vi "ElevatorSim_WouldHitUpperLimit.vi"(10 "Height_Meters":dbl=1.0, 11 "ElevatorSim":T1 {"GearBox"."Kt_NMPerAmp" format="%13.5p"; "GearBox"."Kv_RadPerSecPerVolt" format="%13.5p"; "GearBox"."R_Ohms" format="%13.5p"; "GearBox"."FreeSpeed_RadPerSec" format="%13.5p"; "GearBox"."FreeCurrent_Amps" format="%13.5p"; "GearBox"."StallCurrent_Amps" format="%13.5p"; "GearBox"."StallTorque_NM" format="%13.5p"; "GearBox"."nominalVoltage_Volts" format="%13.5p"}) -> (3 "At HIgh LImit":bool)   [LabVIEW 2019, in "Trajectory_Library.lvlib"]
doc: "Creates a new LINEAR SYSTEM data cluster with the specified values. \n\n\nInputs: \n - XXX -- XXX.\n\nOutputs:\n - XXX -- XXX."
uses:
  LinearSystem_New.vi
  MatBuilder_Create.vi
  MatBuilder_Fill.vi
  MatrixHelper_Zero.vi
  MatrixHelper_CoerceSize.vi
  Trajectory_Library.lvlib
  LINEAR_SYSTEM.ctl
  <vilib>/Analysis/Matrix/Datatypes/RealMatrix.ctl
  <vilib>/Analysis/Matrix/NI_Matrix.lvlib
  DCMOTOR.CTL
  LINEAR_SYSTEM_SIM.ctl
  ELEVATOR_SIM.ctl
panel:
  # "<States, 1>"
  # "<Outputs, 1>"
  # "<Inputs, 1>"
  # "<Outputs, 1>"
  # "<States,States>"
  # "<States,Inputs>"
  # "<Outputs,States>"
  # "<Outputs,Inputs>"
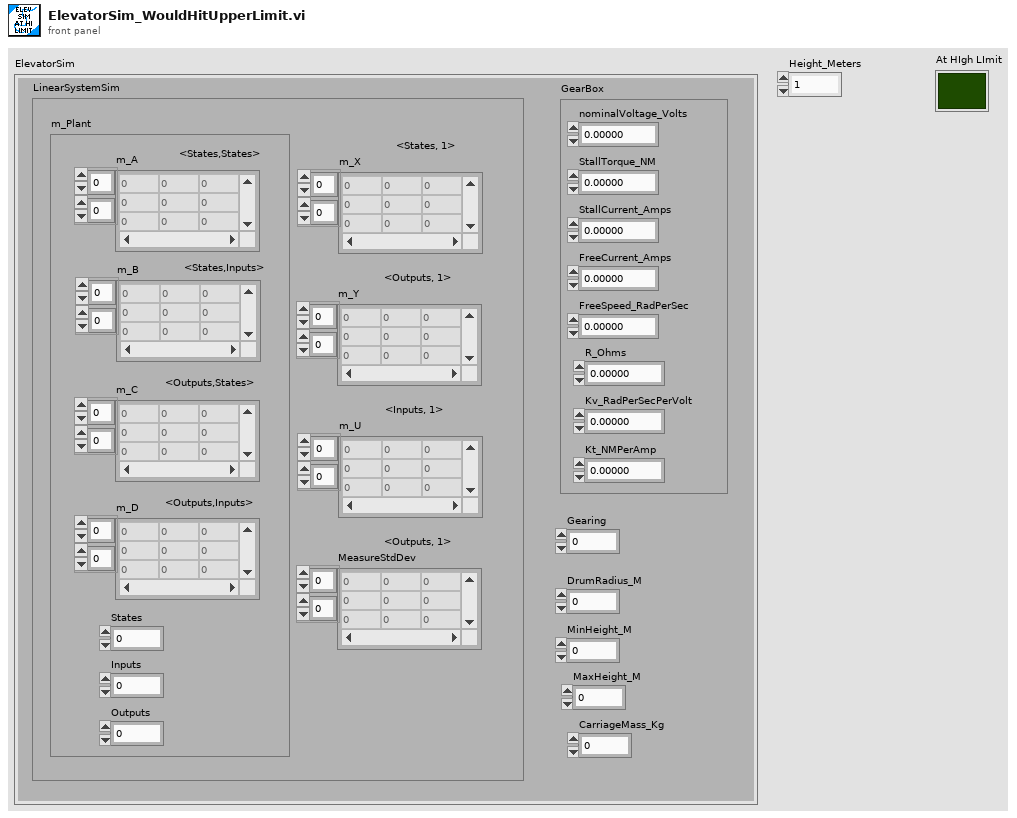
[diagram p1: front panel]
types:
  T1 = typedef "Trajectory_Library.lvlib/ELEVATOR_SIM.ctl" = cluster{"LinearSystemSim":T2, "GearBox":T5, "Gearing":dbl, "DrumRadius_M":dbl, "MinHeight_M":dbl, "MaxHeight_M":dbl, "CarriageMass_Kg":dbl}
  T2 = typedef "Trajectory_Library.lvlib/LINEAR_SYSTEM_SIM.ctl" = cluster{"m_Plant":T3, "m_X":T4, "m_Y":T4, "m_U":T4, "MeasureStdDev":T4}
  T3 = typedef "Trajectory_Library.lvlib/LINEAR_SYSTEM.ctl" = cluster{"m_A":T4, "m_B":T4, "m_C":T4, "m_D":T4, "States":i32, "Inputs":i32, "Outputs":i32}
  T4 = typedef "NI_Matrix.lvlib/RealMatrix.ctl" = dbl[][]
  T5 = typedef "Trajectory_Library.lvlib/DCMOTOR.CTL" = cluster{"nominalVoltage_Volts":dbl, "StallTorque_NM":dbl, "StallCurrent_Amps":dbl, "FreeCurrent_Amps":dbl, "FreeSpeed_RadPerSec":dbl, "R_Ohms":dbl, "Kv_RadPerSecPerVolt":dbl, "Kt_NMPerAmp":dbl}
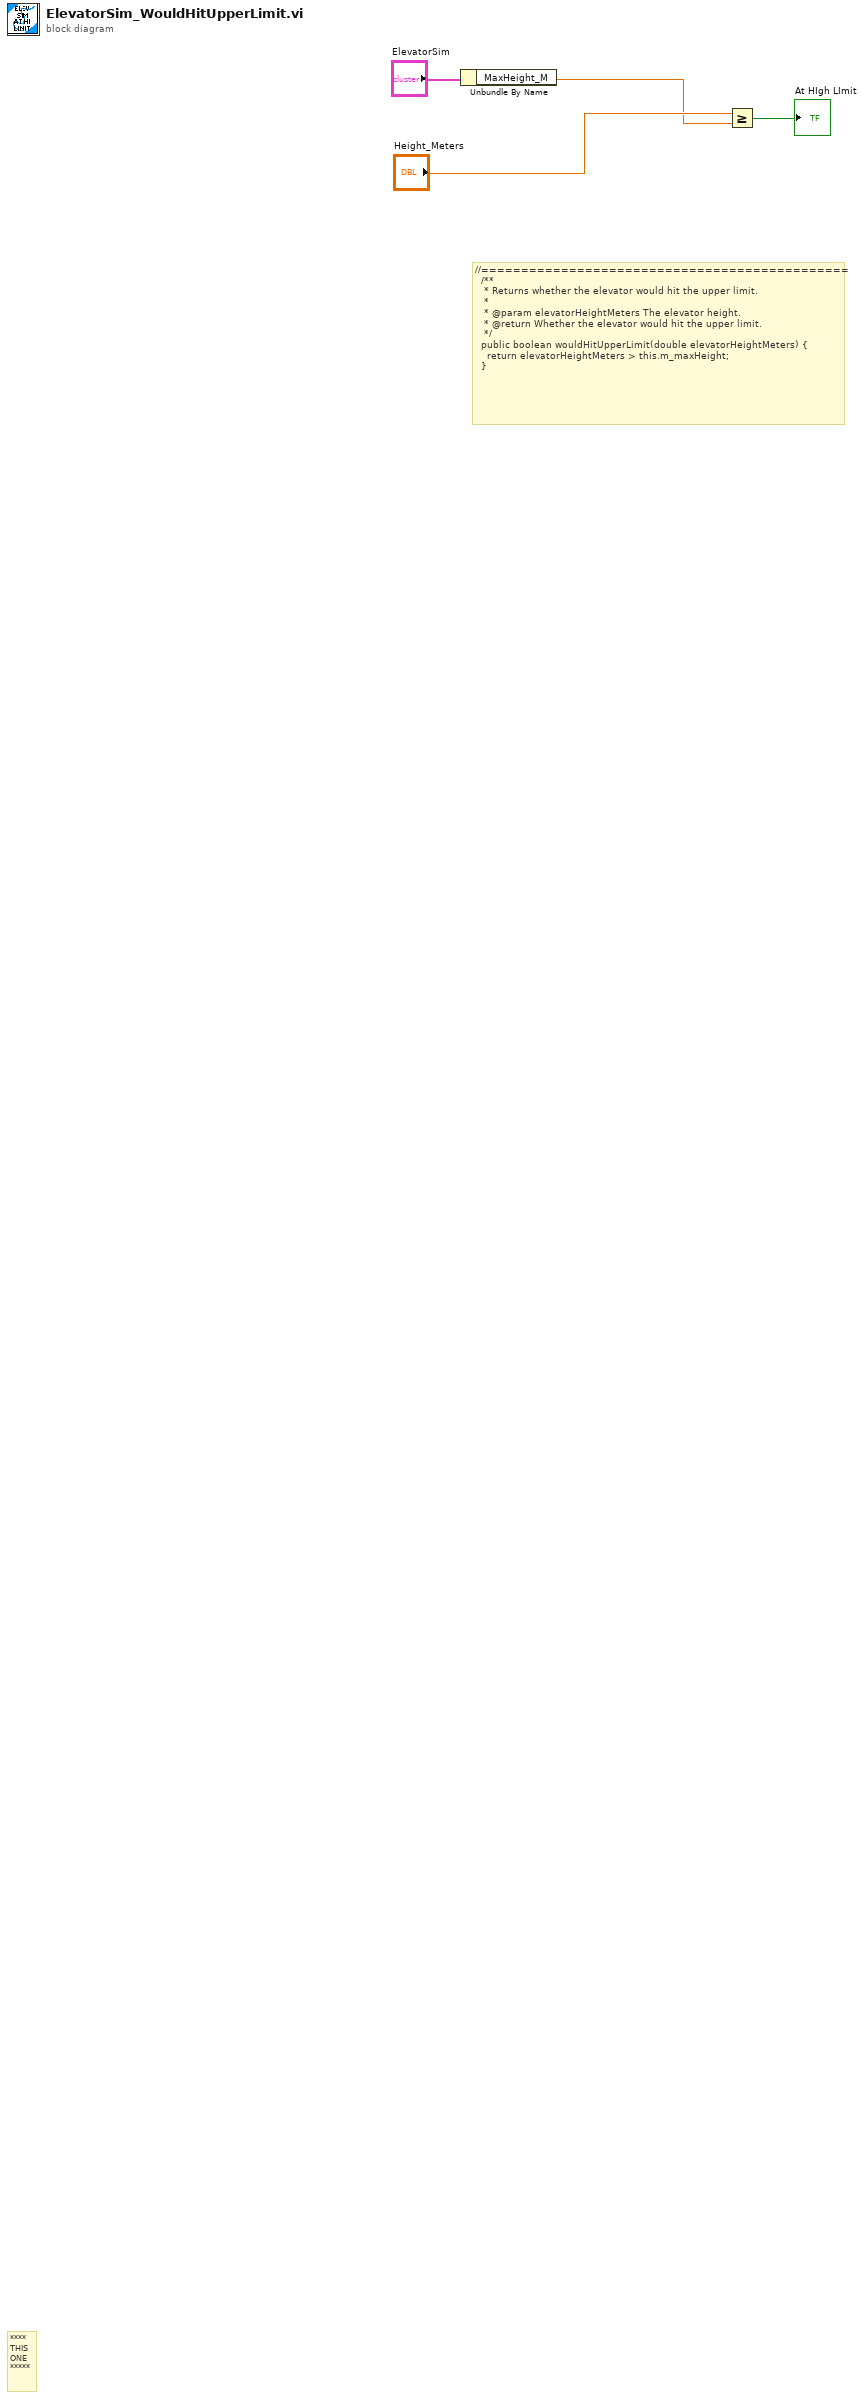
[diagram p0: block diagram]
diagram:
  # "//==============================================\n  /**\n   * Returns whether the elevator would hit the upper limit.\n   *\n   * @param elevatorHeightMeters The elevator height.\n   * @return Whether the elevator would hit the upper limit.\n   */\n  public boolean wouldHitUpperLimit(double elevatorHeightMeters) {\n    return elevatorHeightMeters > this.m_maxHeight;\n  }"
  # "****\nTHIS\nONE\n*****"
  n1 = Unbundle By Name("ElevatorSim") -> ("MaxHeight_M"=w1:dbl)
  n2 = Greater Or Equal?(x="Height_Meters", y=w1) -> (x >= y?=→"At HIgh LImit":bool)
